vi "Check cursor movement.vi"(0 "Display State In":T1, 5 "CursRef":refnum<vi>, 9 "Container State":T2, 11 "error in (no error)":errorcluster) -> (4 "Display State Out":T1, 15 "error out":errorcluster)   [LabVIEW 2014, in "Graph with cursors XControl.xctl"]
uses:
  Graph with cursors XControl.xctl
  <vilib>/_xctls/Container State.ctl
  Graph with cursors State.ctl
  <vilib>/_xctls/XControlSupport.lvlib
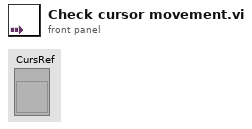
[diagram p1: front panel]
types:
  T1 = typedef "Graph with cursors XControl.xctl/Graph with cursors State.ctl" = cluster{"Cursor names":string[], "Cursor positions":dbl[], "Cursor pairs":i32, "Graph":refnum<vi>, "Prefix":string, "Base path":path}
  T2 = typedef "XControlSupport.lvlib/Container State.ctl" = cluster{"Indicator?":bool, "Run Mode?":bool, " Refnum":refnum<vi>}
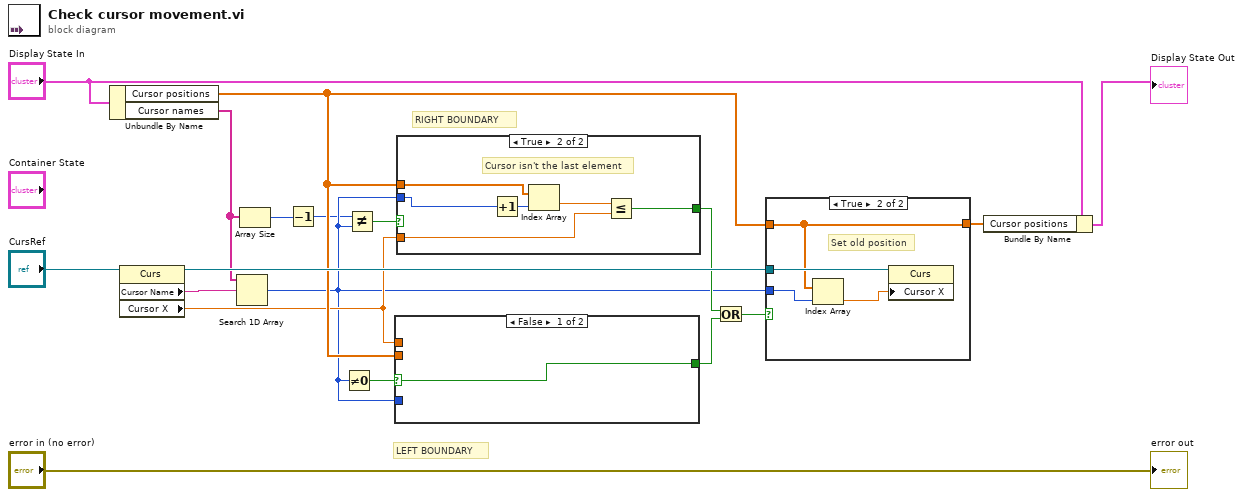
[diagram p0: block diagram]
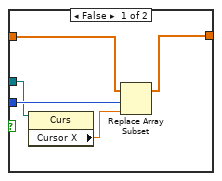
[diagram p2: hidden frame]
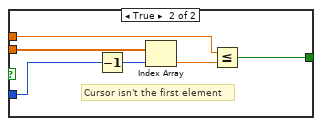
[diagram p4: hidden frame]
diagram:
  # "LEFT BOUNDARY"
  # "RIGHT BOUNDARY"
  n1 = Unbundle By Name("Display State In") -> ("Cursor positions"=w17:dbl[], "Cursor names"=w11:string[])
  n2 = property class="Curs"(reference="CursRef") -> (reference out=w18:refnum<vi>, "Cursor Name"=w15:string, "Cursor X"=w8:dbl)  [unwired: 1 in, 1 out]
  n3 = Search 1D Array(1D array=w11, element=w15) -> (index of element=w2:i32)  [unwired: 1 in]
  n4 = Array Size(array=w11) -> (size(s)=w9:i32)
  n5 = Decrement(x=w9) -> (x-1=w1:i32)
  n6 = Not Equal To 0?(x=w2) -> (x != 0?=w14:bool)
  n7 = Not Equal?(x=w1, y=w2) -> (x != y?=w10:bool)
  n8 = case shown="False" w14 {
    selector: w14 -> [w19 _]
    tunnel: w2 -> [_ w25]
    tunnel: w8 -> [_ w23]
    tunnel: [w19 w21] -> w6
    tunnel: w17 -> [_ w20]
    frame False {
    }
    frame True {
      # "Cursor isn't the first element"
      n9 = Decrement(x=w25) -> (x-1=w24:i32)
      n10 = Index Array(array=w20, index=w24) -> (element=w22:dbl)
      n11 = Less Or Equal?(x=w23, y=w22) -> (x <= y?=w21:bool)
    }
  }
  n12 = case shown="True" w10 {
    selector: w10 -> [w26 _]
    tunnel: [w26 w27] -> w7
    tunnel: w17 -> [_ w31]
    tunnel: w8 -> [_ w28]
    tunnel: w2 -> [_ w30]
    frame False {
      # "Cursor is the last element"
    }
    frame True {
      # "Cursor isn't the last element"
      n13 = Increment(x=w30) -> (x+1=w32:i32)
      n14 = Index Array(array=w31, index=w32) -> (element=w29:dbl)
      n15 = Less Or Equal?(x=w29, y=w28) -> (x <= y?=w27:bool)
    }
  }
  n16 = Or(x=w7, y=w6) -> (x .or. y?=w13:bool)
  n17 = case shown="True" w13 {
    tunnel: w2 -> [w36 w40]
    tunnel: w18 -> [w33 w39]
    tunnel: w17 -> [w35 w38]
    tunnel: [w34 w38] -> w5
    frame False {
      n18 = property class="Curs"(reference=w33) -> ("Cursor X"=w37:dbl)  [unwired: 1 in, 2 out]
      n19 = Replace Array Subset(array=w35, new element=w37, index=w36) -> (w34:dbl[])
    }
    frame True {
      # "Set old position"
      n20 = Index Array(array=w38, index=w40) -> (element=w41:dbl)
      n21 = property class="Curs"(reference=w39, "Cursor X"=w41) -> ()  [unwired: 1 in, 2 out]
    }
  }
  n22 = Bundle By Name(cluster="Display State In", "Cursor positions"=w5) -> (→"Display State Out":T1)
  "error out" <- "error in (no error)"
